vi "Running Average.vi"(8 "Error In":errorcluster, 11 "Async State Vars 2":T1) -> (0 "Error Out":errorcluster, 3 "Async State Vars out":T1)   [LabVIEW 2015, in "Waveform-Processing-Custom-Device Shared.lvlib" / "Running Average.lvlib"]
uses:
  Shared/Running Average/Running Average.lvlib
  Built/Waveform-Processing-Custom-Device/c/Waveform-Processing-Custom-Device Engine Pharlap.llb/Circular Buffer Operations.ctl
  Built/Waveform-Processing-Custom-Device/c/Waveform-Processing-Custom-Device Engine Pharlap.llb/Circular Buffer.lvlib
  Built/Waveform-Processing-Custom-Device/c/Waveform-Processing-Custom-Device Engine Pharlap.llb/Circular Buffer(2D DBL).vi
  <vilib>/Analysis/NI_AALBase.lvlib
  <vilib>/Analysis/baseanly.llb/Mean (DBL).vi
  Types/Async FIFOs.ctl
  Waveform-Processing-Custom-Device Engine.lvlib
  <vilib>/NI Veristand/Custom Device Waveform API/Single Waveform Read (DBL)/Single Waveform Read (DBL).lvclass
  Types/Async State Vars.ctl
  <vilib>/NI Veristand/Custom Device Waveform API/Single Waveform Write (DBL)/Single Waveform Write (DBL).lvclass
  <vilib>/NI Veristand/Custom Device API/Waveform Data Reference.ctl
  <vilib>/NI VeriStand/Custom Device API/Custom Device API.lvlib
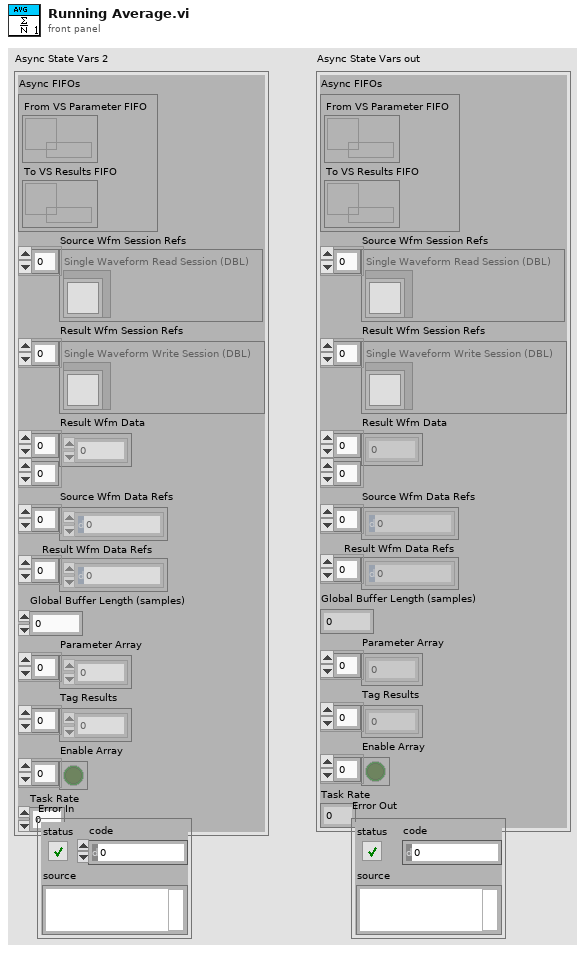
[diagram p1: front panel]
types:
  T1 = typedef "Waveform-Processing-Custom-Device Engine.lvlib/Async State Vars.ctl" = cluster{"Async FIFOs":T2, "Source Wfm Session Refs":refnum<class "Single Waveform Read (DBL).lvclass">[], "Result Wfm Session Refs":refnum<class "Single Waveform Write (DBL).lvclass">[], "Result Wfm Data":dbl[][], "Source Wfm Data Refs":T3[], "Result Wfm Data Refs":T3[], "Global Buffer Length (samples)":dbl, "Parameter Array":dbl[], "Tag Results":dbl[], "Enable Array":bool[], "Task Rate":dbl}
  T2 = typedef "Waveform-Processing-Custom-Device Engine.lvlib/Async FIFOs.ctl" = cluster{"From VS Parameter FIFO":refnum<k33>, "To VS Results FIFO":refnum<k33>}
  T3 = typedef "Custom Device API.lvlib/Waveform Data Reference.ctl" = i32
  T4 = typedef "Circular Buffer.lvlib/Circular Buffer Operations.ctl" = enum16{"Initialize", "Get Backlog", "Write", "Read (continuous)", "Read (most recent)"}
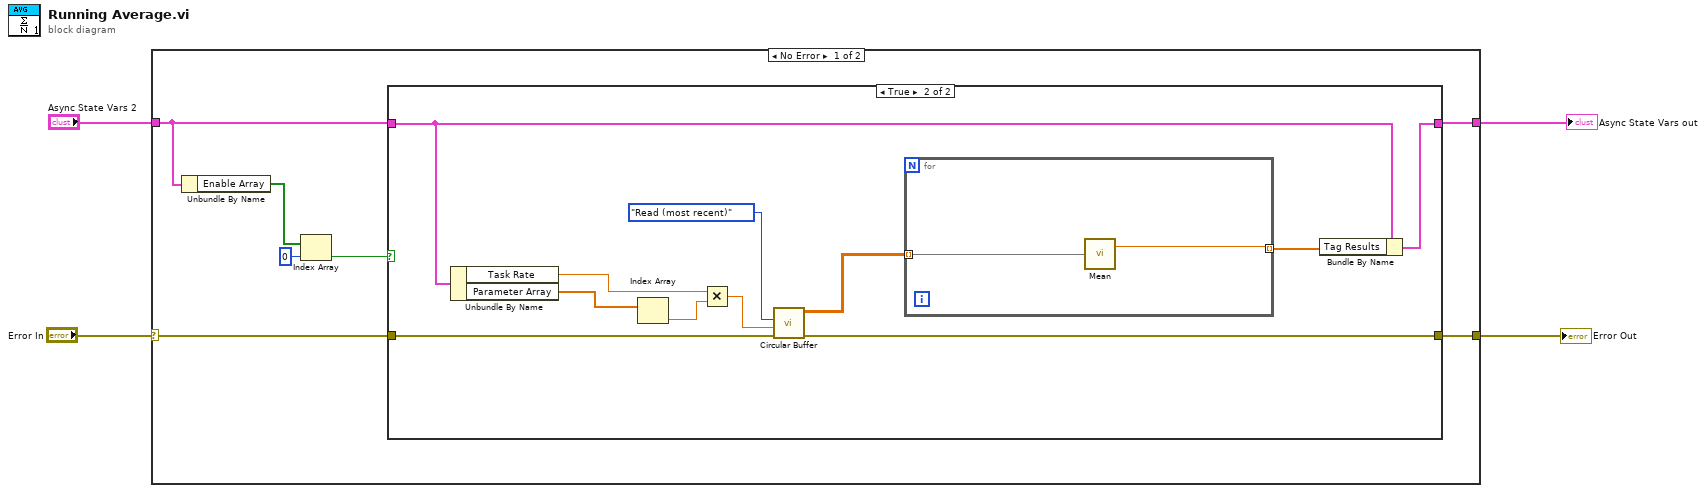
[diagram p0: block diagram]
diagram:
  n1 = case shown="No Error" "Error In" {
    selector: "Error In" -> [w11 w28]
    tunnel: [w10 w28] -> w3
    tunnel: "Async State Vars 2" -> [w8 w27]
    tunnel: [w9 w27] -> w1
    frame No Error {
      n2 = Unbundle By Name(w8) -> ("Enable Array"=w7:bool[])
      n3 = Index Array(array=w7, index=0) -> (element=w6:bool)
      n4 = case shown="True" w6 {
        tunnel: w11 -> [w13 w22]
        tunnel: [w13 w21] -> w10
        tunnel: w8 -> [w12 w20]
        tunnel: [w12 w18] -> w9
        frame False {
        }
        frame True {
          n5 = Unbundle By Name(w20) -> ("Task Rate"=w15:dbl, "Parameter Array"=w17:dbl[])
          n6 = Index Array(array=w17) -> (element=w16:dbl)  [unwired: 1 in]
          n7 = Multiply(x=w15, y=w16) -> (x*y=w14:dbl)
          n8 = call-poly <userlib>:"Circular Buffer.vi"("error in (no error)"=w22, "Read Size"=w14, "Operation"=Circular_Buffer_Operations."Read (most recent)") -> ("error out"=w21:errorcluster, "Data Out"=w23:dbl[][])  [unwired: 5 in, 2 out]
          n9 = for {
            tunnel: w23 -> [w26] mode=indexing
            tunnel: [w25] -> w19 mode=indexing
            n10 = call-poly <vilib>:"Mean.vi"("X"=w26) -> ("mean"=w25:dbl)  [unwired: 1 out]
          }
          n11 = Bundle By Name(cluster=w20, "Tag Results"=w19) -> (w18:T1)
        }
      }
    }
    frame Error {
    }
  }
  "Error Out" <- w3
  "Async State Vars out" <- w1
